vi "3-4 my_LED_step3.vi"() -> ()   [LabVIEW 2014]
doc: "------------------------------------\nAuther: Koji Ohashi\nCopyright (c) 2020 Japan LabVIEW Users Group, Volunteer members.\nThis VI is released under the MIT License.\nhttp://opensource.org/licenses/mit-license.php\n------------------------------------"
panel:
  out "LED Broken":bool
  in  "Continuous Forward Current (mA)":dbl
  out "Current(A)":dbl
  in  "Current Limiting Resistor (ƒ¶)":dbl
  in  "Forward Voltage (V)":dbl min=0.0 step=0.1
  in  "Power-supply voltage (V)":dbl
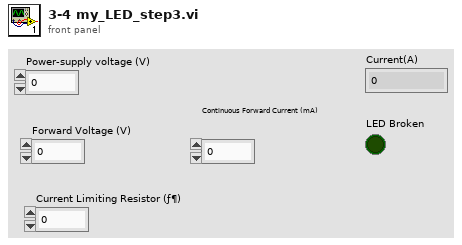
[diagram p1: front panel]
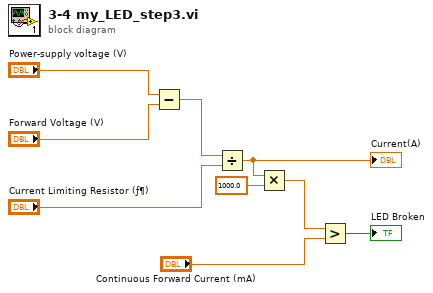
[diagram p0: block diagram]
diagram:
  n1 = Subtract(x="Power-supply voltage (V)", y="Forward Voltage (V)") -> (x-y=w7:dbl)
  n2 = Divide(x=w7, y="Current Limiting Resistor (ƒ¶)") -> (x/y=w3:dbl)
  "Current(A)" <- w3
  n3 = Multiply(x=w3, y=1000.0) -> (x*y=w1:dbl)
  n4 = Greater?(x=w1, y="Continuous Forward Current (mA)") -> (0:→"LED Broken":bool)
